vi "Read Self Q.vi"(8 "error in (no error)":errorcluster, 11 "Engine_Tools in":refnum<class "Engine.lvclass">) -> (0 "error out":errorcluster, 2 "Self Q":refnum<class "Message Enqueuer.lvclass">, 3 "Engine_Tools out":refnum<class "Engine.lvclass">)   [LabVIEW 2023, in "Engine.lvlib" / "Engine.lvclass"]
uses:
  Project/Engine.lvclass
  builds/Engine/Actor Framework.lvlibp/1abvi3w/vi.lib/ActorFramework/Message Enqueuer/Message Enqueuer.lvclass
  Project/Engine.lvclass/Engine.ctl
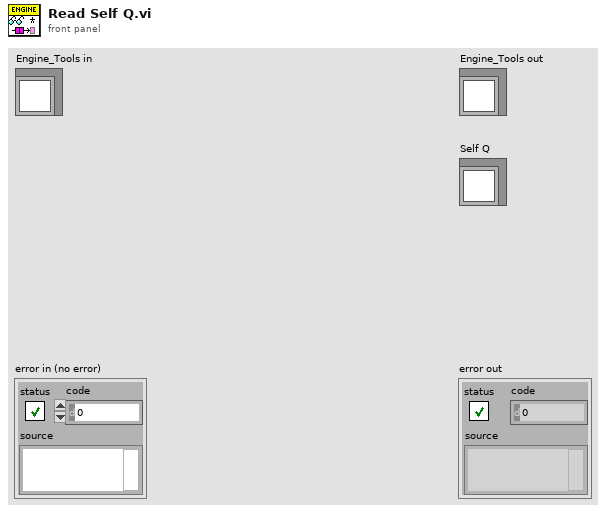
[diagram p1: front panel]
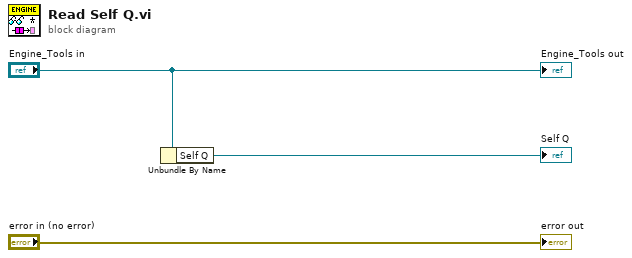
[diagram p0: block diagram]
diagram:
  n1 = Unbundle By Name("Engine_Tools in") -> ("Self Q"=→"Self Q":refnum<class "Message Enqueuer.lvclass">)
  "error out" <- "error in (no error)"
  "Engine_Tools out" <- "Engine_Tools in"
